vi "ODE-PredatorPrey.vi"() -> ()   [LabVIEW 2023]
doc: "This example demonstrates how to use the polymorphic ODE solver in both Formula Sting mode and VI mode. Note that VI mode allows the user to set the values of constants via front panel controls, and the formula is implemented as a call by reference to another VI."
uses:
  <vilib>/Simulation/Utility/Implementation/Shared/SIM Diagram Parameters.ctl
  <vilib>/Simulation/Implementation/Shared/SIM Continuous Solvers.ctl
  <vilib>/gmath/ode.llb/ODE Solver formula string.vi
  <vilib>/gmath/ode.llb/ODE Solver main.vi
  <vilib>/gmath/NI_Gmath.lvlib
panel:
  out "Population vs. Time":cluster{"times":dbl[], dbl[]}[](graph)
  in  "Stop":bool
  in  "Constants":cluster{"a":dbl, "b":dbl, "c":dbl, "d":dbl}={"a"=2.0, "b"=0.01, "c"=1.0, "d"=0.010000000000000009}
  in  "Initial Conditions for variables (x1, x2)":dbl[](array[numeric])=[300.0, 50.0]
  in  "Formula String Parameters":T1={"ODE Right Hand Side"=["a*x1-b*x1*x2", "-c*x2+d*x1*x2"], "X (name of variables)"=["x1", "x2"], "time"="t"}
  # "Overview: This example demonstrates how to use the polymorphic ODE solver in both Formula String mode and VI mode.\nRequirements: LabVIEW Full Development System\nInstructions: \n1. Run the VI.\n2. Modify the input parameters of the ODE solver(s).\n3. Click Stop to stop the VI."
  # "This example demonstrates how to use the polymorphic ODE solver in both Formula String mode and VI mode.  Note that VI mode allows for setting constant values via front panel controls, and the formula is passed by reference from a separate VI.\n\nThis separate VI contains the formula in LabVIEW code of the Predator-Prey ODE system model:\n\ndx1/dt = ax1 - bx1x2\ndx2/dt = -cx2 + dx1x2\n\nwhere x1 is the population of the prey and x2 is the population of the predators."
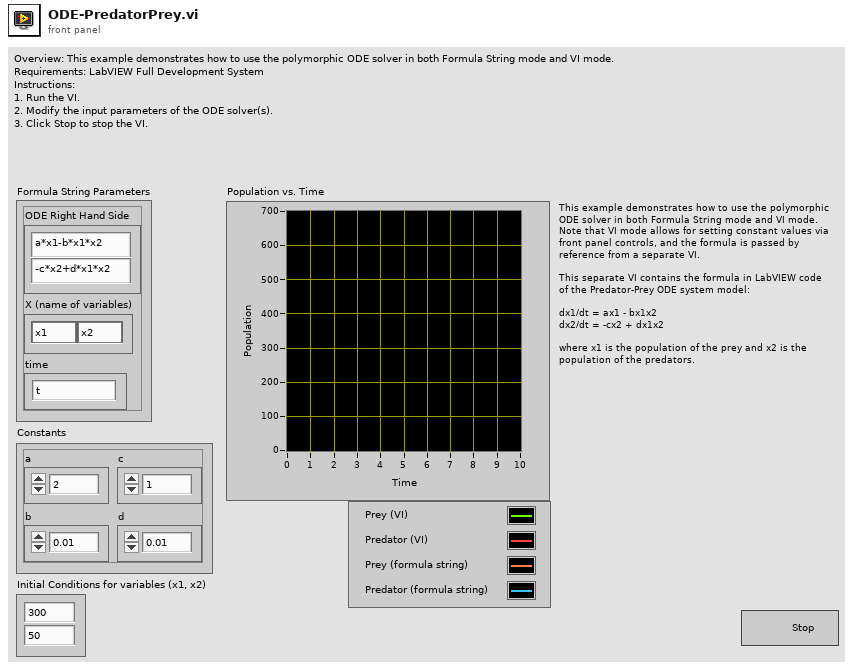
[diagram p1: front panel]
types:
  T1 = cluster{"ODE Right Hand Side":string[], "X (name of variables)":string[], "time":string}
  T2 = typedef "SIM Diagram Parameters.ctl" = cluster{"Initial Time":dbl, "Final Time":dbl, "Time Step":dbl, "Absolute Tolerance":dbl, "Relative Tolerance":dbl, "Continuous Solver":T3, "Discrete Time Step":dbl, "Minimum Time Step":dbl, "Maximum Time Step":dbl, "Initial Time Step":dbl}
  T3 = typedef "SIM Continuous Solvers.ctl" = enum16{"Runge-Kutta 1 (Euler)", "Runge-Kutta 2", "Runge-Kutta 3", "Runge-Kutta 4", "Runge-Kutta 23 (variable)", "Runge-Kutta 45 (variable)", "BDF (variable)", "Adams-Moulton (variable)", "Rosenbrock (variable)", "Discrete States Only"}
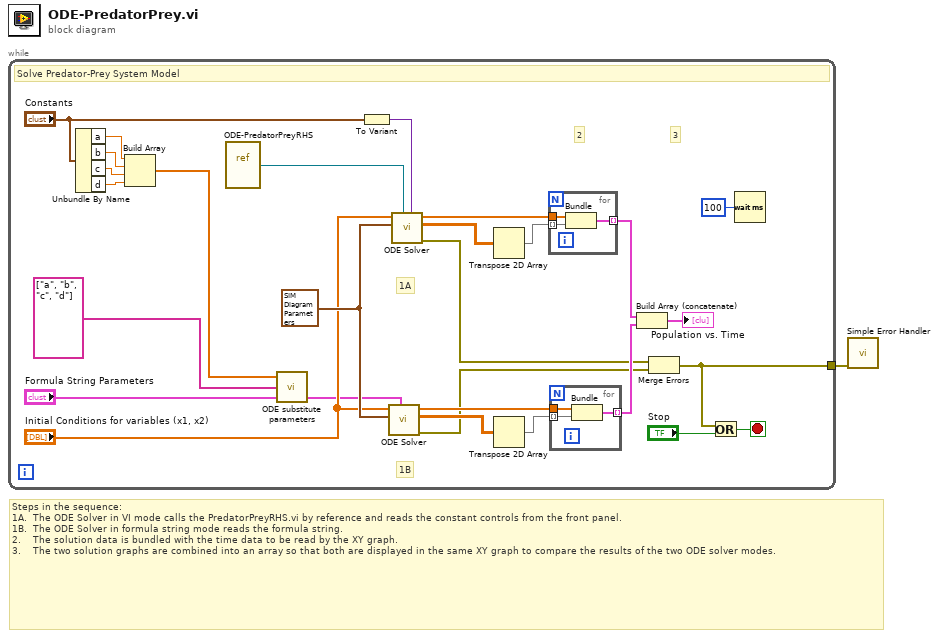
[diagram p0: block diagram]
diagram:
  # "Steps in the sequence:\n1A.  The ODE Solver in VI mode calls the PredatorPreyRHS.vi by reference and reads the constant controls from the front panel.\n1B.  The ODE Solver in formula string mode reads the formula string.\n2.    The solution data is bundled with the time data to be read by the XY graph.\n3.    The two solution graphs are combined into an array so that both are displayed in the same XY graph to compare the results of the two ODE solver modes."
  n1 = while {
    tunnel: [w2] -> w1
    stop <- w5 stop-if-true
    w25 = T2 {"Initial Time"=0.0, "Final Time"=10.0, "Time Step"=0.1, "Absolute Tolerance"=0.001, "Relative Tolerance"=1e-06, "Continuous Solver"=enum."Adams-Moulton (variable)", "Discrete Time Step"=2.0, "Minimum Time Step"=1e-06, "Maximum Time Step"=1.0, "Initial Time Step"=0.01} ("Simulation Parameters")
    # "3"
    # "1B"
    # "2"
    # "1A"
    # "Solve Predator-Prey System Model"
    n2 = Unbundle By Name("Constants") -> ("a"=w14:dbl, "b"=w13:dbl, "c"=w12:dbl, "d"=w11:dbl)
    n3 = Build Array(w14, w13, w12, w11) -> (w10:dbl[])
    n4 = vi-ref "ODE-PredatorPreyRHS.vi"() -> ("vi reference"=w29:refnum<vi>)
    n5 = call "ODE substitute parameters.vi"("Formula String Parameters"="Formula String Parameters", "parameters"=string[] ["a", "b", "c", "d"], "values"=w10) -> ("Formula String Parameters with substitutions"=w7:T1)  [unwired: 2 out]
    n6 = To Variant(anything="Constants") -> (Variant=w17:variant)
    n7 = call-poly <vilib>:"ODE Solver.vi"("ODE RHS"=w7, "simulation parameters"=w25, "x0"="Initial Conditions for variables (x1, x2)") -> ("error out"=w4:errorcluster, "outputs"=w20:dbl[][], "times"=w24:dbl[])  [unwired: 1 in, 5 out]
    n8 = call-poly <vilib>:"ODE Solver.vi"("data"=w17, "ODE F(X,t)"=w29, "simulation parameters"=w25, "x0"="Initial Conditions for variables (x1, x2)") -> ("error out"=w3:errorcluster, "outputs"=w26:dbl[][], "times"=w27:dbl[])  [unwired: 1 in, 4 out]
    n9 = Transpose 2D Array(2D array=w26) -> (transposed array=w28:dbl[][])
    n10 = Transpose 2D Array(2D array=w20) -> (transposed array=w21:dbl[][])
    n11 = for {
      tunnel: w28 -> [w35] mode=indexing
      tunnel: w27 -> [w34]
      tunnel: [w33] -> w19 mode=indexing
      n12 = Bundle("times"=w34, w35) -> (w33:cluster{"times":dbl[], dbl[]})  [unwired: 1 out]
    }
    n13 = for {
      tunnel: w21 -> [w32] mode=indexing
      tunnel: w24 -> [w31]
      tunnel: [w30] -> w23 mode=indexing
      n14 = Bundle("times"=w31, w32) -> (w30:cluster{"times":dbl[], dbl[]})  [unwired: 1 out]
    }
    n15 = Build Array (concatenate)(w19, w23) -> (→"Population vs. Time":cluster{"times":dbl[], dbl[]}[])
    n16 = Merge Errors(w3, w4) -> (w2:errorcluster)
    n17 = Or(x=w2, y="Stop") -> (x .or. y?=w5:bool)
    n18 = Wait (ms)(milliseconds to wait=u32 100 ("millisecond multiple")) -> ()  [unwired: 1 out]
  }
  n19 = call <vilib>:"Simple Error Handler.vi"("error in (no error)"=w1) -> ()  [unwired: 4 in, 5 out]
